vi "Filter 1D Array.vi"(10 "Input":string[](array[string]), 11 "Selector array":bool[](array[boolean])=[TRUE, TRUE, TRUE, TRUE, TRUE, TRUE, TRUE, TRUE, TRUE, TRUE, TRUE, FALSE, TRUE, FALSE, TRUE, FALSE, TRUE, FALSE, TRUE, FALSE, TRUE, FALSE, TRUE, FALSE, TRUE, FALSE, TRUE, FALSE, TRUE, FALSE, TRUE, TRUE]) -> (0 "True":string[](array[string]), 3 "False":string[](array[string]))   [LabVIEW 2025]
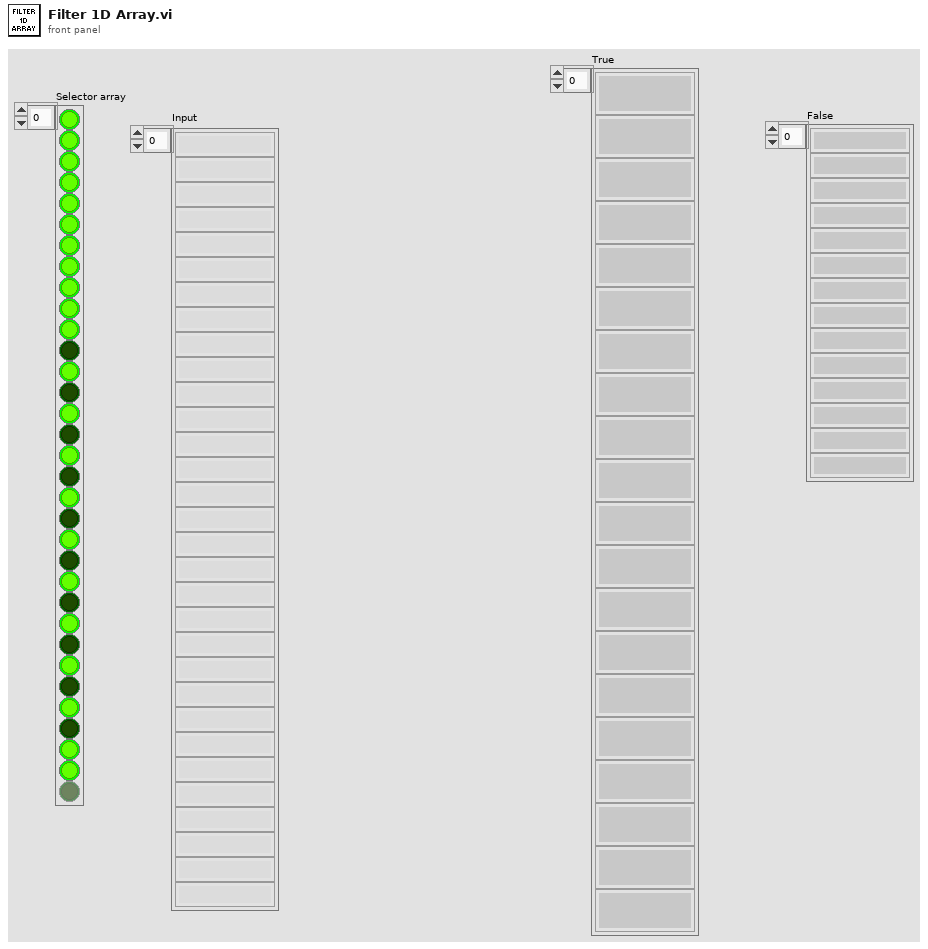
[diagram p1: front panel]
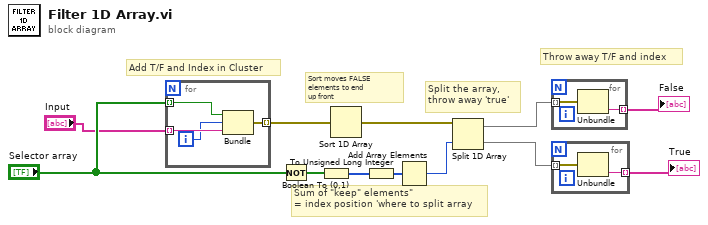
[diagram p0: block diagram]
diagram:
  # "Add T/F and Index in Cluster"
  # "Throw away T/F and index"
  # "Sum of \"keep\" elements\"\n= index position 'where to split array"
  # "Split the array,\nthrow away 'true'"
  # "Sort moves FALSE elements to end\nup front"
  n1 = for {
    tunnel: "Input" -> [w14] mode=indexing
    tunnel: "Selector array" -> [w15] mode=indexing
    tunnel: [w16] -> w3 mode=indexing
    i -> [w13]
    n2 = Bundle(w15, w13, "String"=w14) -> (w16:cluster{bool, i32, "String":string})  [unwired: 1 in]
  }
  n3 = Not(x="Selector array") -> (.not. x?=w11:bool[])
  n4 = Boolean To (0,1)(Boolean=w11) -> (0, 1=w9:i16[])
  n5 = Sort 1D Array(array=w3) -> (sorted array=w4:cluster{bool, i32, "String":string}[])
  n6 = To Unsigned Long Integer(number=w9) -> (unsigned 32bit integer=w8:u32[])
  n7 = Add Array Elements(numeric array=w8) -> (sum=w12:u32)
  n8 = Split 1D Array(array=w4, index=w12) -> (first subarray=w2:cluster{bool, i32, "String":string}[], second subarray=w7:cluster{bool, i32, "String":string}[])
  n9 = for {
    tunnel: w2 -> [w18] mode=indexing
    tunnel: [w17] -> w10 mode=indexing
    n10 = Unbundle(w18) -> ("String"=w17:string)  [unwired: 2 out]
  }
  "False" <- w10
  n11 = for {
    tunnel: w7 -> [w20] mode=indexing
    tunnel: [w19] -> w6 mode=indexing
    n12 = Unbundle(w20) -> ("String"=w19:string)  [unwired: 2 out]
  }
  "True" <- w6
